vi "gc-zyklus.vi"() -> ()   [LabVIEW 2010]
panel:
  out "Zyklus Nr.":i32
  in  "Positionen (1-6)":i32[](array[numeric])=[1, 3, 5, 2]
  out "Anzahl der Zustände (Mpos.-Ventil)":i32
  out "Position":i32
  in  "Werte der Zustände":i32[](array[numeric])=[1, 3, 5, 2]
  in  "Längen der Zustände (s)":i32[](array[numeric])=[1, 3, 5, 2]
  out "Anzahl der Zustände (z.B. MFC)":i32
  out "Länge des Zustandes \"i\" (s)":i32
  out "Wert des Zustandes \"i\"":i32
  out "Sequenz Nr.":i32
  out "Aktuelle Zeit":timestamp
  in  "(Sequenz wird zu Ende geführt)":bool
  # "Gerät im Chromatographie-Zyklus, z.B. MFC"
  # "Multipositionsventil"
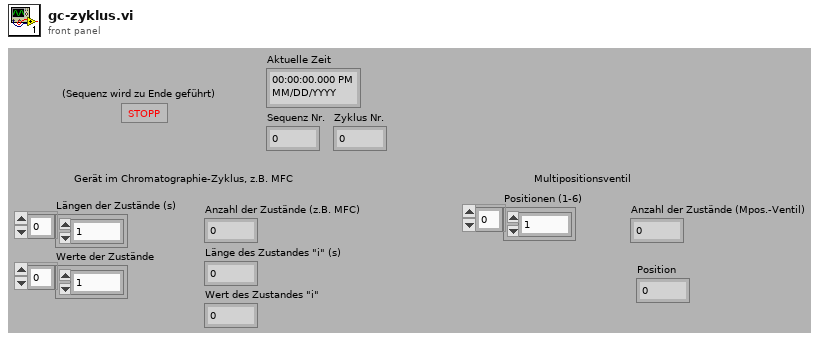
[diagram p1: front panel]
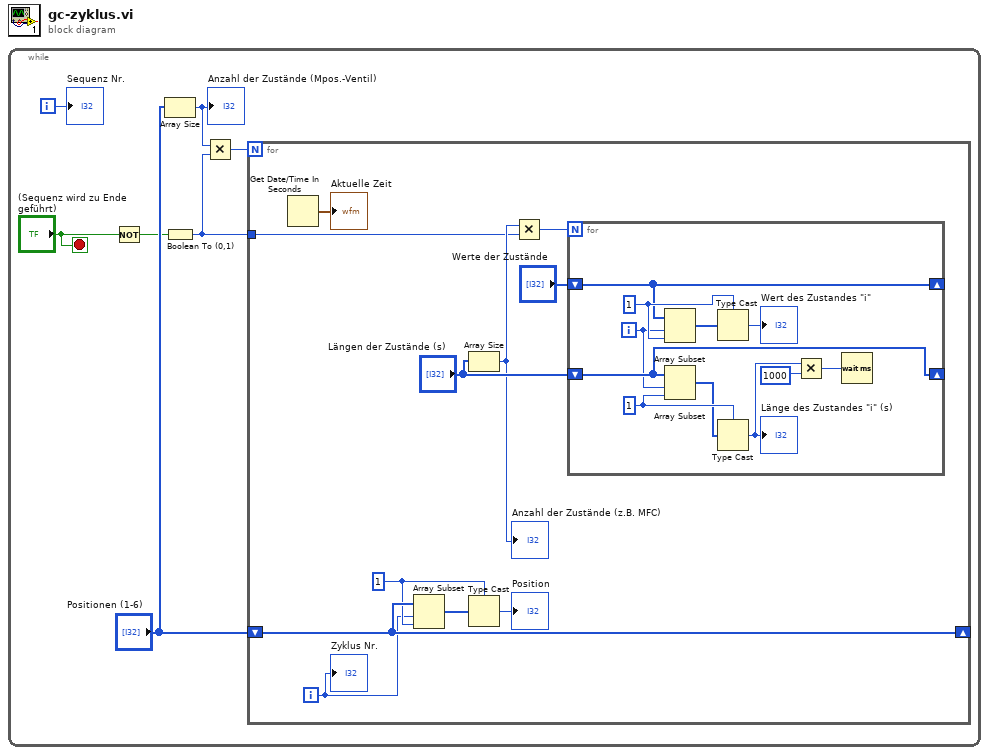
[diagram p0: block diagram]
diagram:
  n1 = while {
    i -> [w6]
    stop <- "(Sequenz wird zu Ende geführt)" stop-if-true
    n2 = Not(x="(Sequenz wird zu Ende geführt)") -> (.not. x?=w3:bool)
    n3 = Array Size(array="Positionen (1-6)") -> (size(s)=w5:i32)
    "Anzahl der Zustände (Mpos.-Ventil)" <- w5
    n4 = Boolean To (0,1)(Boolean=w3) -> (0, 1=w1:i16)
    n5 = Multiply(x=w5, y=w1) -> (x*y=w2:i32)
    n6 = for {
      N: w2 -> [_]
      shift-right: [w18] -> _
      shift-left: "Positionen (1-6)" -> [w18]
      tunnel: w1 -> [w9]
      i -> [w14]
      w17 = 1 ("Länge")
      n7 = Get Date/Time In Seconds() -> (seconds since 1Jan1904=→"Aktuelle Zeit":timestamp)
      n8 = Array Subset(array=w18, index=w14, length=w17) -> (w16:i32[])
      n9 = Array Size(array="Längen der Zustände (s)") -> (size(s)=w10:i32)
      "Anzahl der Zustände (z.B. MFC)" <- w10
      n10 = Type Cast(type=w17, x=w16) -> (*(type *) &x=→"Position":i32)
      n11 = Multiply(x=w10, y=w9) -> (x*y=w8:i32)
      n12 = for {
        N: w8 -> [_]
        shift-right: [w28] -> _
        shift-left: "Längen der Zustände (s)" -> [w28]
        shift-right: [w19] -> _
        shift-left: "Werte der Zustände" -> [w19]
        i -> [w20]
        w23 = 1 ("Länge")
        w27 = 1 ("Länge")
        n13 = Array Subset(array=w19, index=w20, length=w23) -> (w22:i32[])
        n14 = Array Subset(array=w28, index=w20, length=w27) -> (w26:i32[])
        n15 = Type Cast(type=w23, x=w22) -> (*(type *) &x=→"Wert des Zustandes \"i\"":i32)
        n16 = Type Cast(type=w27, x=w26) -> (*(type *) &x=w25:i32)
        "Länge des Zustandes \"i\" (s)" <- w25
        n17 = Multiply(x=w25, y=1000) -> (x*y=w24:i32)
        n18 = Wait (ms)(milliseconds to wait=w24) -> ()  [unwired: 1 out]
      }
      "Zyklus Nr." <- w14
    }
    "Sequenz Nr." <- w6
  }
